vi "Actor Core.vi"(8 "error in":errorcluster, 11 "Monitor Window in":refnum<class "Classic Monitor.lvclass">) -> (0 "error out":errorcluster, 3 "Actor out":refnum<class "Actor.lvclass">)   [LabVIEW 2017, in "MGI-Monitored Actor.lvlib" / "Classic Monitor.lvclass"]
doc: "(<B>Filename</B>: Actor Framework.lvlib:Actor.lvclass:Actor Core.vi)\n\nReceives messages to the actor, reacts to them, and initiates any error handling that may shut the actor down.\n\nDescendant classes may override this VI to append parallel tasks for the actor to complete while it handles messages. Overrides use the Call Parent Method node."
uses:
  Classic Monitor.lvclass
  C:/Program Files (x86)/National Instruments/LabVIEW 2017/vi.lib/ActorFramework/Actor/Actor.lvclass
  <vilib>/ActorFramework/Actor/Actor.lvclass
  monitored-actor-core/Source/Monitor Data/Monitor Data.lvclass
  <vilib>/ActorFramework/Message Enqueuer/Message Enqueuer.lvclass
  <vilib>/ActorFramework/Actor/Actor.lvclass/Actor.ctl
  <vilib>/ActorFramework/Message Enqueuer/Message Enqueuer.lvclass/Message Enqueuer.ctl
  Classic Monitor.lvclass/Classic Monitor.ctl
  <vilib>/ActorFramework/Time-Delayed Send Message/Time-Delay Override Options.ctl
  <vilib>/ActorFramework/Stop Msg/Stop Msg.lvclass/Stop Msg.ctl
  Orphan Detector/Orphan Detector/Orphan Detector.lvclass
  <vilib>/ActorFramework/Message Enqueuer/Init from Existing Queue.vi
  <vilib>/ActorFramework/Message Enqueuer/Enqueue.vi
  <vilib>/ActorFramework/Message Enqueuer/Enqueue Critical.vi
  <vilib>/ActorFramework/Stop Msg/Stop Msg.lvclass
  C:/Program Files (x86)/National Instruments/LabVIEW 2017/vi.lib/ActorFramework/Message/Message.lvclass
  monitored-actor-core/Source/Actor Monitor/Actor Monitor Messages/Ping Actor Msg/Ping Actor Msg.lvclass
  <vilib>/ActorFramework/Message Priority Queue/Priority Enqueue.vi
  monitored-actor-core/Source/Actor Monitor/Actor Monitor/Actor Monitor.lvclass
  Classic Monitor Messages/Log Messages Msg/Log Messages Msg.lvclass
  monitored-actor-core/Source/Actor Monitor/Actor Monitor Messages/Manually Remove Actor Msg/Manually Remove Actor Msg.lvclass
panel:
  in  "Monitored Actors":string[](tree)
  in  "Stop Actor":bool
  in  "Show Actor Core":bool
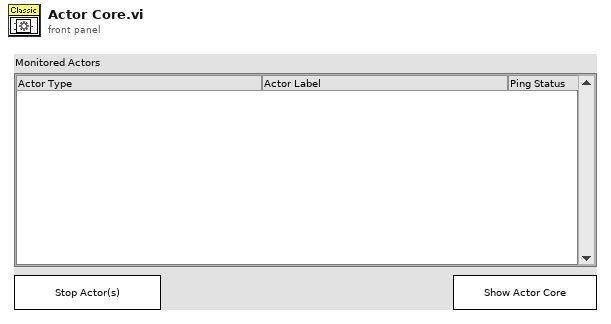
[diagram p1: front panel]
types:
  T1 = cluster{"Monitor Data":refnum<class "Monitor Data.lvclass">, "Changed Actor Q":refnum<class "Message Enqueuer.lvclass">}
  T2 = enum32{"Invalid", "Standard", "Closed", "Hidden", "Minimized", "Maximized"}
  T3 = cluster{"left":i16, "top":i16, "right":i16, "bottom":i16}
  T4 = typedef "Time-Delay Override Options.ctl" = enum16{"Send next copy now", "Skip next scheduled copy", "Send next copy now and stop all further copies", "Stop all further copies"}
  T5 = enum8{"Enabled", "Disabled", "Disabled and Grayed Out"}
  T6 = typedef "LVRectTypeDef.ctl" = cluster{"Left":i16, "Top":i16, "Right":i16, "Bottom":i16}
  T7 = typedef "LVPoint32TypeDef.ctl" = cluster{"Horizontal":i32, "Vertical":i32}
  T8 = typedef "MGI-Monitored Actor Core.lvlib/Monitor Data.lvclass/Actor Data.ctl" = cluster{"Actor Type":string, "Actor Cores":string[], "Self":refnum<class "Message Enqueuer.lvclass">, "Caller":refnum<class "Message Enqueuer.lvclass">, "Actor Label":string, "Last Ping":dbl}
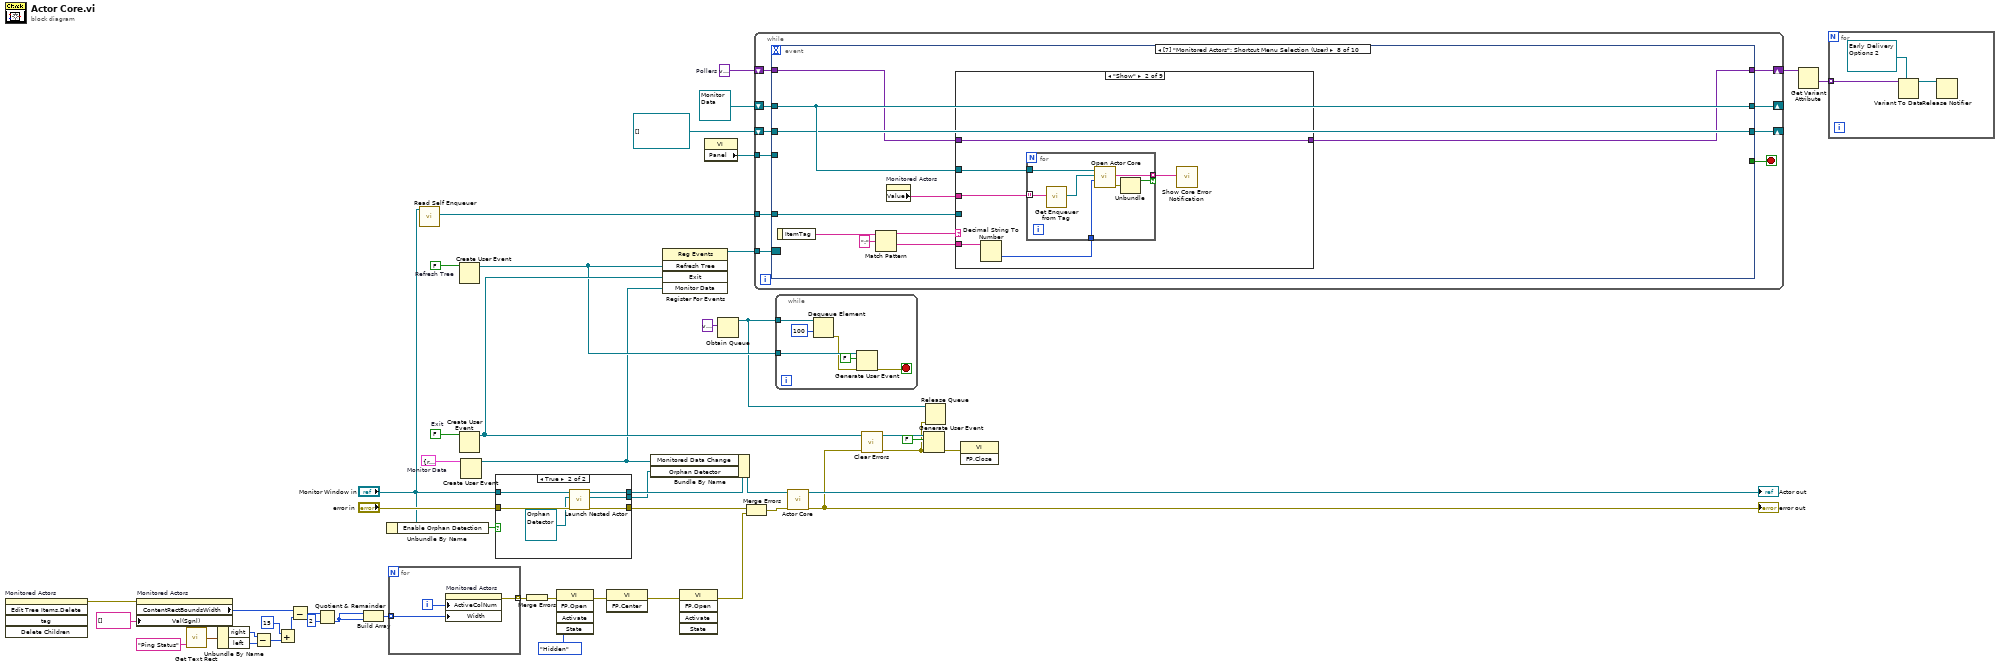
[diagram p0: block diagram]
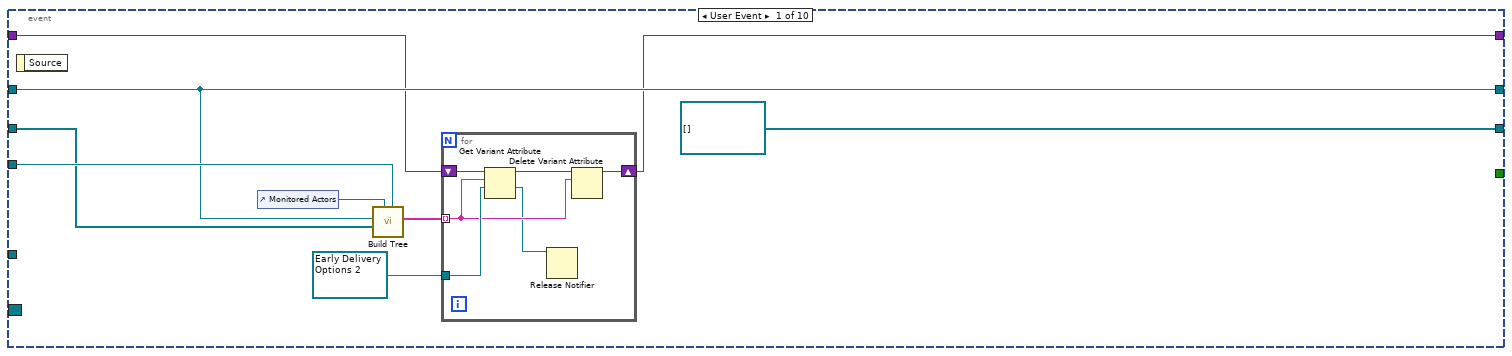
[diagram p3: hidden frame]
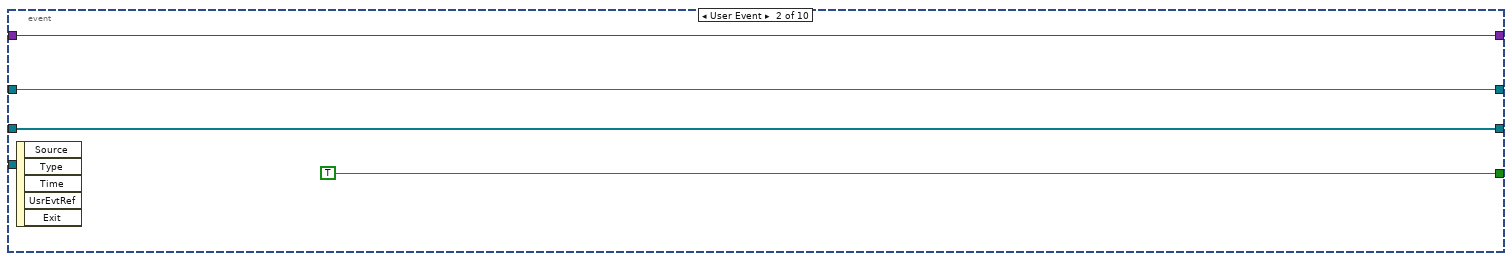
[diagram p4: hidden frame]
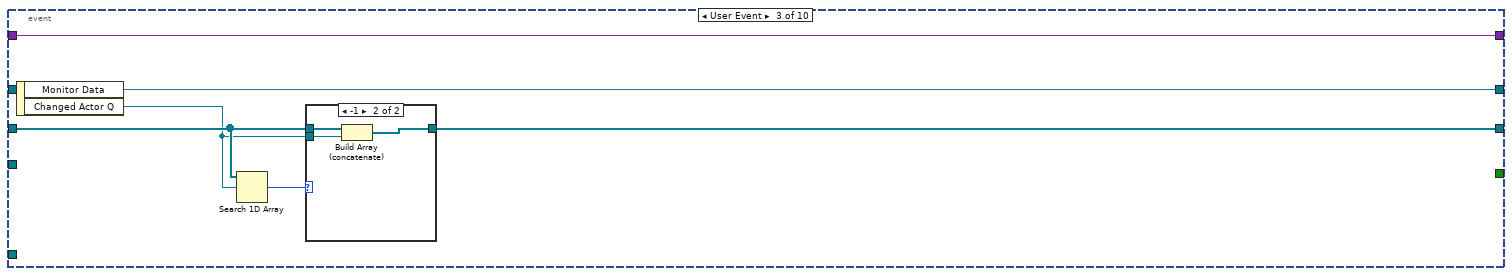
[diagram p5: hidden frame]
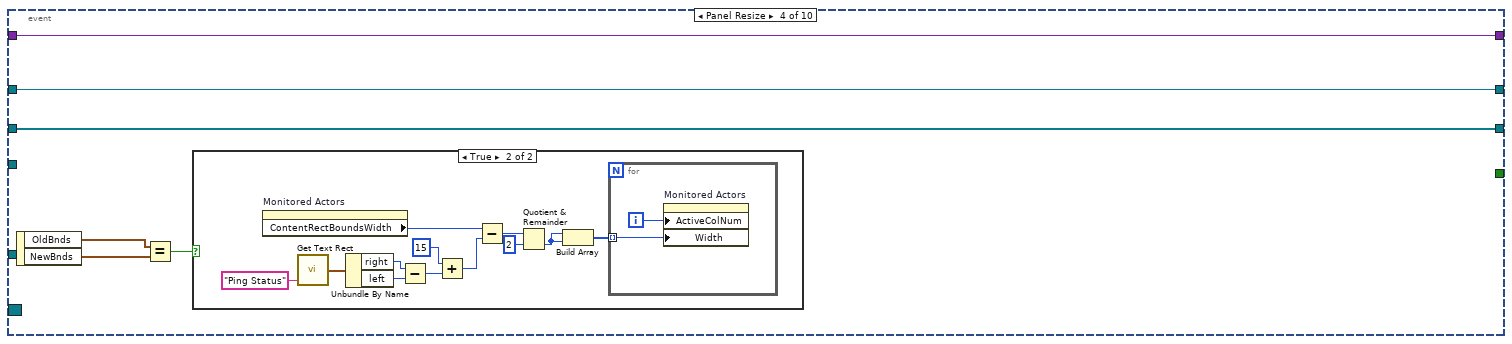
[diagram p7: hidden frame]
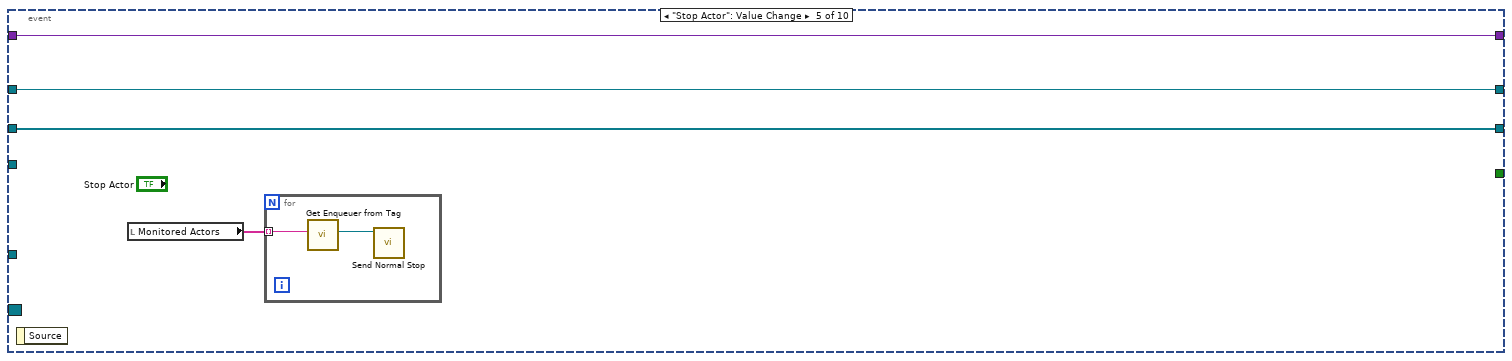
[diagram p9: hidden frame]
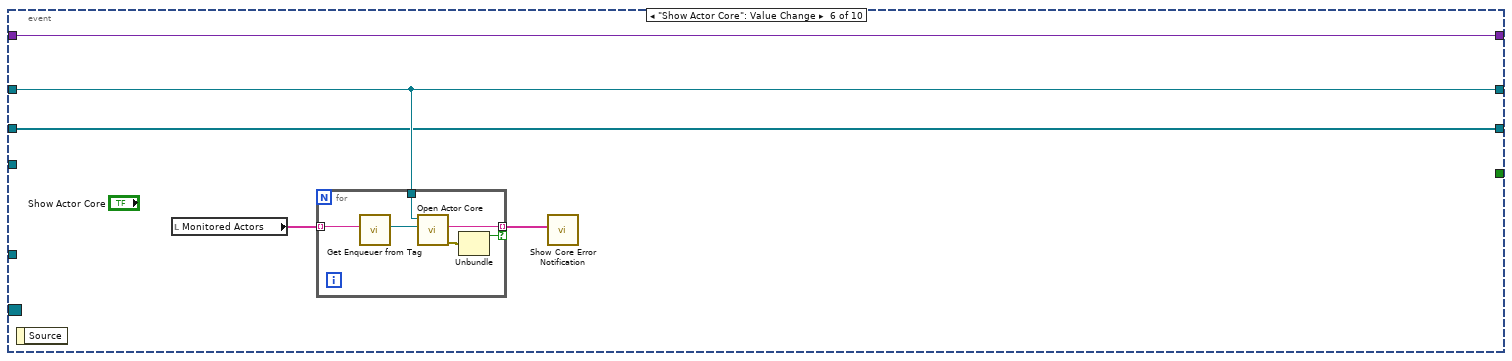
[diagram p10: hidden frame]
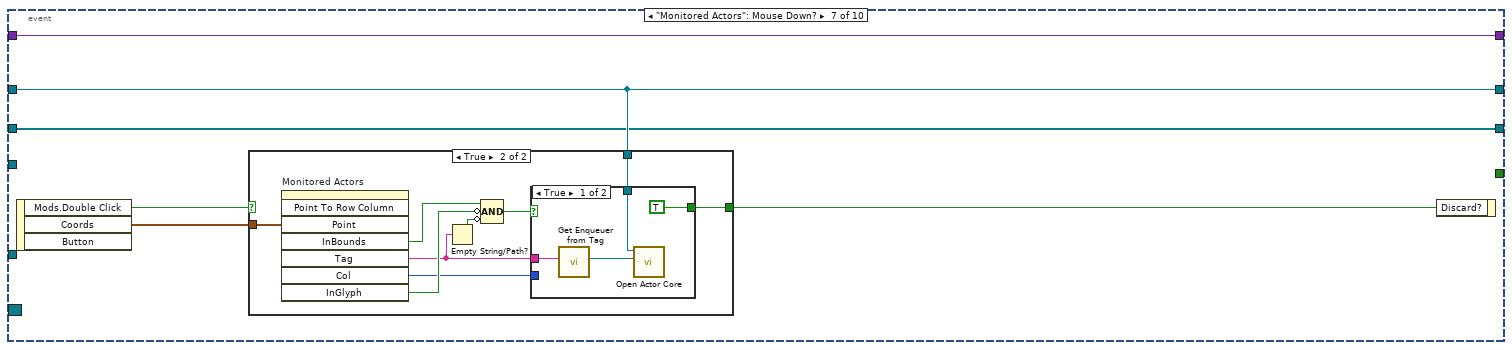
[diagram p11: hidden frame]
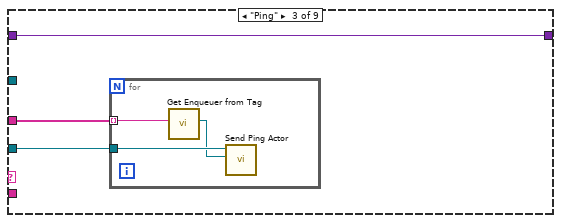
[diagram p15: hidden frame]
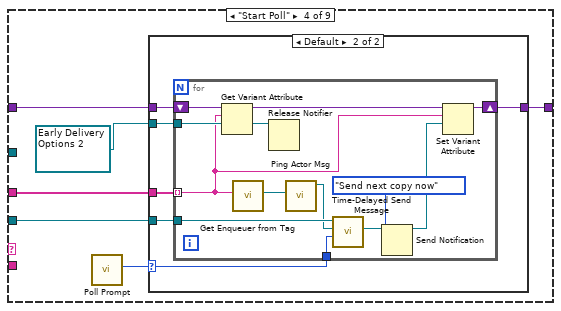
[diagram p16: hidden frame]
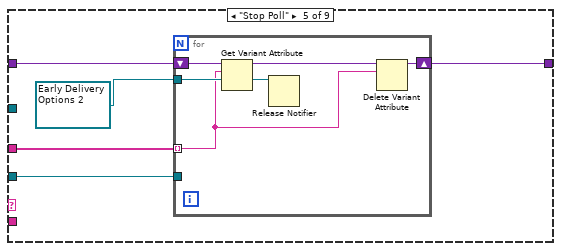
[diagram p18: hidden frame]
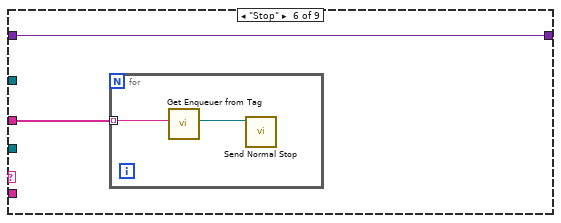
[diagram p19: hidden frame]
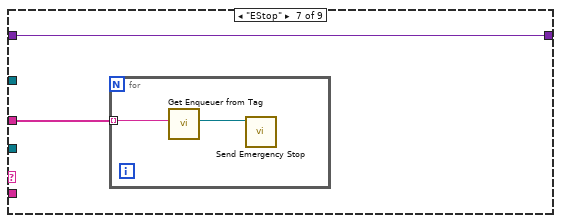
[diagram p20: hidden frame]
diagram:
  w6 = variant  # Pollers
  w17 = T1 {"Monitor Data"=refnum, "Changed Actor Q"=refnum}  # Monitor Data
  w22 = FALSE  # Refresh Tree
  w34 = FALSE  # Exit
  n1 = invoke on="Monitored Actors" class="Tree (strict)" method="Edit Tree Items.Delete"() -> (error out=w13:errorcluster)  [unwired: 5 in, 4 out]
  n2 = property on="Monitored Actors" class="Tree (strict)"(error in=w13, "Val(Sgnl)"=string[] [] ("Value (Signaling)")) -> ("ContentRectBoundsWidth"=w47:i32)  [unwired: 1 in, 2 out]
  n3 = call <vilib>:"Get Text Rect.vi"("text"="Ping Status") -> ("rect"=w45:T3)  [unwired: 8 in]
  n4 = Unbundle By Name(w45) -> ("right"=w44:i16, "left"=w43:i16)
  n5 = Subtract(x=w44, y=w43) -> (x-y=w42:i16)
  n6 = Add(x=i16 15, y=w42) -> (x+y=w39:i16)
  n7 = Subtract(x=w47, y=w39) -> (x-y=w41:i32)
  n8 = Quotient & Remainder(x=w41, y=2) -> (floor(x/y)=w37:i32)  [unwired: 1 out]
  n9 = Build Array(w37, w37) -> (w36:i32[])
  n10 = Unbundle By Name("Monitor Window in") -> ("Enable Orphan Detection"=w7:bool)
  n11 = for {
    tunnel: w36 -> [w51] mode=indexing
    tunnel: [w50] -> w27 mode=indexing
    i -> [w52]
    n12 = property on="Monitored Actors" class="Tree (strict)"("ActiveColNum"=w52, "Width"=w51) -> (error out=w50:errorcluster)  [unwired: 2 in, 1 out]
  }
  n13 = call <vilib>:"Read Self Enqueuer.vi"("Actor"="Monitor Window in") -> ("Self Enqueuer"=w28:refnum<class "Message Enqueuer.lvclass">)  [unwired: 10 in]
  n14 = Create User Event(user event datatype=w22) -> (user event=w21:refnum<user-event>)  [unwired: 1 in, 1 out]
  n15 = Create User Event(user event datatype=w34) -> (user event=w33:refnum<user-event>)  [unwired: 1 in, 1 out]
  n16 = Create User Event(user event datatype=w17) -> (user event=w16:refnum<user-event>)  [unwired: 1 in, 1 out]
  n17 = case shown="True" w7 {
    tunnel: "error in" -> [w53 w56]
    tunnel: [w53 w57] -> w12
    tunnel: [w54 w59] -> w11
    tunnel: "Monitor Window in" -> [w54 w60]
    tunnel: [_ w58] -> w10
    frame False {
    }
    frame True {
      n18 = call <vilib>:"Launch Nested Actor.vi"("error in (no error)"=w56, "Nested Actor"=refnum<class "Orphan Detector.lvclass"> refnum ("Classic Monitor.lvlib:Orphan Detector.lvclass"), "Caller Actor in"=w60) -> ("error out"=w57:errorcluster, "Nested Actor's Enqueuer"=w58:refnum<class "Message Enqueuer.lvclass">, "Caller Actor out"=w59:refnum<class "Classic Monitor.lvclass">)  [unwired: 6 in]
    }
  }
  n19 = Merge Errors(w27) -> (w25:errorcluster)
  n20 = invoke class="VI" method="FP.Open"(error in=w25, "State"=T2."Hidden") -> (error out=w26:errorcluster)  [unwired: 3 in, 4 out]
  n21 = invoke class="VI" method="FP.Center"(error in=w26) -> (error out=w24:errorcluster)  [unwired: 2 in, 2 out]
  n22 = Bundle By Name(cluster=w11, "Monitored Data Change"=w16, "Orphan Detector"=w10) -> (w31:refnum<class "Classic Monitor.lvclass">)
  n23 = register-events(w21, w33, w16) -> (reference out=w35:refnum<event-registration>)  [unwired: 2 in, 1 out]
  n24 = invoke class="VI" method="FP.Open"(error in=w24) -> (error out=w1:errorcluster)  [unwired: 4 in, 4 out]
  n25 = property class="VI"() -> ("Panel"=w29:refnum<vi>)  [unwired: 2 in, 2 out]
  n26 = Obtain Queue(element data type=variant) -> (queue out=w18:refnum<queue>)  [unwired: 4 in, 2 out]
  n27 = Merge Errors(w12, w1) -> (w2:errorcluster)
  n28 = while {
    tunnel: w35 -> [w70]
    shift-right: [w68] -> _
    shift-left: refnum<class "Monitor Data.lvclass"> refnum ("Monitor Data") -> [w67]
    tunnel: w29 -> [w66]
    tunnel: w28 -> [w65]
    shift-right: [w64] -> _
    shift-left: refnum<class "Message Enqueuer.lvclass">[] [] -> [w63]
    shift-right: [w62] -> w5
    shift-left: w6 -> [w61]
    stop <- w69 stop-if-true
    n29 = event shown="[7] \"Monitored Actors\": Shortcut Menu Selection (User)" {
      selector: w70 -> [_ _ _ _ _ _ _ _ _ _]
      dyn-events: _ -> [_ _ _ _ _ _ _ _ _ _]
      timeout: _ -> [_ _ _ _ _ _ _ _ _ _]
      tunnel: [_ TRUE _ _ _ _ _ _ _ _] -> w69
      tunnel: [w78 w88 w95 w105 w123 w129 w142 w165 w253 w255] -> w68
      tunnel: w67 -> [w78 w88 _ w105 w123 w129 w142 w165 w253 w255]
      tunnel: w66 -> [w79 _ _ _ _ _ _ _ _ _]
      tunnel: w65 -> [_ _ _ _ _ _ _ w163 _ _]
      tunnel: [refnum<class "Message Enqueuer.lvclass">[] [] w87 w94 w101 w121 w128 w138 w162 w254 w276] -> w64
      tunnel: w63 -> [w76 w87 w93 w101 w121 w128 w138 w162 w254 w276]
      tunnel: [w71 w86 w90 w100 w120 w126 w137 w160 w247 w269] -> w62
      tunnel: w61 -> [w72 w86 w90 w100 w120 w126 w137 w161 w247 w269]
      event User Event {
        w73 = refnum<notifier> refnum items=["Send next copy now", "Skip next scheduled copy", "Send next copy now and stop all further copies", "Stop all further copies"] ("Delivery Notifier")
        n30 = event-data() -> ()  [unwired: 1 in, 1 out]
        n31 = control-ref of="Monitored Actors"() -> (w77:refnum<vi>)
        n32 = call "Build Tree.vi"("Panel"=w79, "Tree"=w77, "Changed Actors"=w76, "Monitor Data"=w78) -> ("Stopped Actors"=w74:string[])  [unwired: 7 in]
        n33 = for {
          tunnel: w74 -> [w82] mode=indexing
          shift-right: [w81] -> w71
          shift-left: w72 -> [w85]
          tunnel: w73 -> [w84]
          n34 = Get Variant Attribute(Variant=w85, name=w82, default value (empty Variant)=w84) -> (duplicate Variant=w83:variant, value=w80:refnum<notifier>)  [unwired: 1 in, 2 out]
          n35 = Release Notifier(notifier=w80) -> ()  [unwired: 2 in, 3 out]
          n36 = Delete Variant Attribute(6:w82, 7:w83) -> (3:w81:variant)  [unwired: 1 in, 2 out]
        }
      }
      event User Event {
        n37 = event-data() -> ()  [unwired: 1 in, 5 out]
      }
      event User Event {
        n38 = event-data() -> ("Monitor Data"=w95:refnum<class "Monitor Data.lvclass">, "Changed Actor Q"=w92:refnum<class "Message Enqueuer.lvclass">)  [unwired: 1 in]
        n39 = Search 1D Array(1D array=w93, element=w92) -> (index of element=w91:i32)  [unwired: 1 in]
        n40 = case shown="-1" w91 {
          tunnel: [w96 w99] -> w94
          tunnel: w93 -> [w96 w98]
          tunnel: w92 -> [_ w97]
          frame Default {
          }
          frame -1 {
            n41 = Build Array (concatenate)(w98, w97) -> (w99:refnum<class "Message Enqueuer.lvclass">[])
          }
        }
      }
      event Panel Resize {
        n42 = event-data() -> ("OldBnds"=w104:T6, "NewBnds"=w103:T6)  [unwired: 1 in]
        n43 = Equal?(x=w104, y=w103) -> (x = y?=w102:bool)
        n44 = case shown="True" w102 {
          frame False {
          }
          frame True {
            n45 = property on="Monitored Actors" class="Tree (strict)"() -> ("ContentRectBoundsWidth"=w106:i32)  [unwired: 2 in, 2 out]
            n46 = call <vilib>:"Get Text Rect.vi"("text"="Ping Status") -> ("rect"=w108:T3)  [unwired: 8 in]
            n47 = Unbundle By Name(w108) -> ("right"=w109:i16, "left"=w110:i16)
            n48 = Subtract(x=w109, y=w110) -> (x-y=w111:i16)
            n49 = Add(x=i16 15, y=w111) -> (x+y=w114:i16)
            n50 = Subtract(x=w106, y=w114) -> (x-y=w112:i32)
            n51 = Quotient & Remainder(x=w112, y=2) -> (floor(x/y)=w116:i32)  [unwired: 1 out]
            n52 = Build Array(w116, w116) -> (w117:i32[])
            n53 = for {
              tunnel: w117 -> [w118] mode=indexing
              i -> [w119]
              n54 = property on="Monitored Actors" class="Tree (strict)"("ActiveColNum"=w119, "Width"=w118) -> ()  [unwired: 2 in, 2 out]
            }
          }
        }
      }
      event "Stop Actor": Value Change {
        n55 = event-data() -> ()  [unwired: 1 in, 1 out]
        n56 = local read "Monitored Actors"() -> (w122:string[])
        n57 = for {
          tunnel: w122 -> [w125] mode=indexing
          n58 = call "Get Enqueuer from Tag.vi"("Tag"=w125) -> ("Enqueuer"=w124:refnum<class "Message Enqueuer.lvclass">)  [unwired: 10 in]
          n59 = call <vilib>:"Send Normal Stop.vi"("Message Enqueuer"=w124) -> ()  [unwired: 10 in, 1 out]
        }
      }
      event "Show Actor Core": Value Change {
        n60 = event-data() -> ()  [unwired: 1 in, 1 out]
        n61 = local read "Monitored Actors"() -> (w130:string[])
        n62 = for {
          tunnel: w130 -> [w136] mode=indexing
          tunnel: w129 -> [w135]
          tunnel: [w133] -> w127 mode=indexing if=w131
          n63 = call "Get Enqueuer from Tag.vi"("Tag"=w136) -> ("Enqueuer"=w134:refnum<class "Message Enqueuer.lvclass">)  [unwired: 10 in]
          n64 = call "Open Actor Core.vi"("Actor's Self Q"=w134, "Monitor Data"=w135) -> ("error out"=w132:errorcluster, "Actor Core VI"=w133:string)  [unwired: 8 in]
          n65 = Unbundle(w132) -> ("status"=w131:bool)  [unwired: 2 out]
        }
        n66 = call "Show Core Error Notification.vi"("Error VIs"=w127) -> ()  [unwired: 11 in]
      }
      event "Monitored Actors": Mouse Down? {
        n67 = event-data() -> ("Mods.Double Click"=w141:bool, "Coords"=w140:T7)  [unwired: 1 in, 1 out]
        n68 = case shown="True" w141 {
          tunnel: w142 -> [_ w151]
          tunnel: w140 -> [_ w150]
          tunnel: [_ w147] -> w139
          frame False {
          }
          frame True {
            n69 = invoke on="Monitored Actors" class="Tree (strict)" method="Point To Row Column"("Point"=w150) -> ("InBounds"=w149:bool, "Tag"=w144:string, "Col"=w143:i32, "InGlyph"=w148:bool)  [unwired: 7 in, 4 out]
            n70 = Empty String/Path?(string/path=w144) -> (empty?=w145:bool)
            n71 = Compound Arithmetic op=AND(w149, invert w148, invert w145) -> (w146:bool)
            n72 = case shown="True" w146 {
              tunnel: w151 -> [w153 _]
              tunnel: [TRUE _] -> w147
              tunnel: w144 -> [w155 _]
              tunnel: w143 -> [_ _]
              frame True {
                n73 = call "Get Enqueuer from Tag.vi"("Tag"=w155) -> ("Enqueuer"=w152:refnum<class "Message Enqueuer.lvclass">)  [unwired: 10 in]
                n74 = call "Open Actor Core.vi"("Actor's Self Q"=w152, "Monitor Data"=w153) -> ()  [unwired: 8 in, 2 out]
              }
              frame False {
              }
            }
          }
        }
        n75 = event-data("Discard?"=w139) -> ()  [unwired: 1 in, 1 out]
      }
      event "Monitored Actors": Shortcut Menu Selection (User) {
        n76 = event-data() -> ("ItemTag"=w159:string)  [unwired: 1 in]
        n77 = Match Pattern(string=w159, regular expression=":") -> (before substring=w158:string, after substring=w156:string)  [unwired: 1 in, 2 out]
        n78 = property on="Monitored Actors" class="Tree (strict)"() -> ("Value"=w164:string[])  [unwired: 2 in, 2 out]
        n79 = case shown="\"Show\"" w158 {
          tunnel: w165 -> [_ w171 _ _ _ _ _ _ _]
          tunnel: w164 -> [_ w172 w182 w191 w216 w224 w228 w235 w243]
          tunnel: w163 -> [_ _ w181 w190 w215 _ _ w234 w242]
          tunnel: w161 -> [w166 w169 w180 w189 w214 w223 w227 w233 w241]
          tunnel: [w166 w169 w180 w188 w213 w223 w227 w233 w241] -> w160
          tunnel: w156 -> [_ w168 _ _ _ _ _ _ _]
          frame Default {
          }
          frame "Show" {
            n80 = Decimal String To Number(string=w168) -> (number=w167:i32)  [unwired: 2 in, 1 out]
            n81 = for {
              tunnel: w172 -> [w179] mode=indexing
              tunnel: w171 -> [w178]
              tunnel: [w176] -> w170 mode=indexing if=w174
              tunnel: w167 -> [w173]
              n82 = call "Get Enqueuer from Tag.vi"("Tag"=w179) -> ("Enqueuer"=w177:refnum<class "Message Enqueuer.lvclass">)  [unwired: 10 in]
              n83 = call "Open Actor Core.vi"("Core Index (0)"=w173, "Actor's Self Q"=w177, "Monitor Data"=w178) -> ("error out"=w175:errorcluster, "Actor Core VI"=w176:string)  [unwired: 7 in]
              n84 = Unbundle(w175) -> ("status"=w174:bool)  [unwired: 2 out]
            }
            n85 = call "Show Core Error Notification.vi"("Error VIs"=w170) -> ()  [unwired: 11 in]
          }
          frame "Ping" {
            n86 = for {
              tunnel: w182 -> [w185] mode=indexing
              tunnel: w181 -> [w184]
              n87 = call "Get Enqueuer from Tag.vi"("Tag"=w185) -> ("Enqueuer"=w183:refnum<class "Message Enqueuer.lvclass">)  [unwired: 10 in]
              n88 = call "Send Ping Actor.vi"("Actor"=w183, "Message Enqueuer in"=w184) -> ()  [unwired: 8 in, 2 out]
            }
          }
          frame "Start Poll" {
            w187 = refnum<notifier> refnum items=["Send next copy now", "Skip next scheduled copy", "Send next copy now and stop all further copies", "Stop all further copies"] ("Delivery Notifier")
            n89 = call "Poll Prompt.vi"() -> ("Period"=w186:i32)  [unwired: 10 in, 1 out]
            n90 = case shown="Default" w186 {
              selector: w186 -> [_ w193]
              tunnel: w191 -> [_ w198]
              tunnel: w190 -> [_ w197]
              tunnel: w189 -> [w192 w196]
              tunnel: [w192 w195] -> w188
              tunnel: w187 -> [_ w194]
              frame -1 {
              }
              frame Default {
                n91 = for {
                  tunnel: w198 -> [w202] mode=indexing
                  tunnel: w197 -> [w211]
                  shift-right: [w204] -> w195
                  shift-left: w196 -> [w208]
                  tunnel: w194 -> [w206]
                  tunnel: w193 -> [w201]
                  n92 = Get Variant Attribute(Variant=w208, name=w202, default value (empty Variant)=w206) -> (duplicate Variant=w207:variant, value=w205:refnum<notifier>)  [unwired: 1 in, 2 out]
                  n93 = call "Get Enqueuer from Tag.vi"("Tag"=w202) -> ("Enqueuer"=w210:refnum<class "Message Enqueuer.lvclass">)  [unwired: 10 in]
                  n94 = Release Notifier(notifier=w205) -> ()  [unwired: 2 in, 3 out]
                  n95 = call "Ping Actor Msg.vi"("Actor"=w210) -> ("Ping Actor Msg out"=w209:refnum<class "Ping Actor Msg.lvclass">)  [unwired: 9 in, 1 out]
                  n96 = call <vilib>:"Time-Delayed Send Message.vi"("Milliseconds To Wait"=w201, "Message"=w209, "Message Enqueuer"=w211) -> ("Delivery Notifier"=w203:refnum<notifier>)  [unwired: 7 in, 1 out]
                  n97 = Send Notification(notification=Time-Delay_Override_Options."Send next copy now", notifier=w203) -> (notifier out=w200:refnum<notifier>)  [unwired: 1 in, 1 out]
                  n98 = Set Variant Attribute(Variant=w207, name=w202, value=w200) -> (Variant out=w204:variant)  [unwired: 1 in, 2 out]
                }
              }
            }
          }
          frame "Stop Poll" {
            w212 = refnum<notifier> refnum items=["Send next copy now", "Skip next scheduled copy", "Send next copy now and stop all further copies", "Stop all further copies"] ("Delivery Notifier")
            n99 = for {
              tunnel: w216 -> [w217] mode=indexing
              tunnel: w215 -> [_]
              shift-right: [w218] -> w213
              shift-left: w214 -> [w222]
              tunnel: w212 -> [w220]
              n100 = Get Variant Attribute(Variant=w222, name=w217, default value (empty Variant)=w220) -> (duplicate Variant=w221:variant, value=w219:refnum<notifier>)  [unwired: 1 in, 2 out]
              n101 = Release Notifier(notifier=w219) -> ()  [unwired: 2 in, 3 out]
              n102 = Delete Variant Attribute(6:w217, 7:w221) -> (3:w218:variant)  [unwired: 1 in, 2 out]
            }
          }
          frame "Stop" {
            n103 = for {
              tunnel: w224 -> [w226] mode=indexing
              n104 = call "Get Enqueuer from Tag.vi"("Tag"=w226) -> ("Enqueuer"=w225:refnum<class "Message Enqueuer.lvclass">)  [unwired: 10 in]
              n105 = call <vilib>:"Send Normal Stop.vi"("Message Enqueuer"=w225) -> ()  [unwired: 10 in, 1 out]
            }
          }
          frame "EStop" {
            n106 = for {
              tunnel: w228 -> [w230] mode=indexing
              n107 = call "Get Enqueuer from Tag.vi"("Tag"=w230) -> ("Enqueuer"=w229:refnum<class "Message Enqueuer.lvclass">)  [unwired: 10 in]
              n108 = call <vilib>:"Send Emergency Stop.vi"("Message Enqueuer"=w229) -> ()  [unwired: 10 in, 1 out]
            }
          }
          frame "Remove" {
            n109 = Two Button Dialog(message="Warning: Manually removing actors from list can lead to inconsitancies between the monitor and the actual state.\n\n Only do this if you're sure the actor has been aborted manually.") -> (T button?=w231:bool)  [unwired: 2 in]
            n110 = case shown="True" w231 {
              tunnel: w235 -> [_ w237]
              tunnel: w234 -> [_ w236]
              frame False {
              }
              frame True {
                n111 = for {
                  tunnel: w237 -> [w240] mode=indexing
                  tunnel: w236 -> [w238]
                  n112 = call "Get Enqueuer from Tag.vi"("Tag"=w240) -> ("Enqueuer"=w239:refnum<class "Message Enqueuer.lvclass">)  [unwired: 10 in]
                  n113 = call "Send Manually Remove Actor.vi"("Actor's Q"=w239, "Message Enqueuer in"=w238) -> ()  [unwired: 8 in, 2 out]
                }
              }
            }
          }
          frame "Logging" {
            n114 = for {
              tunnel: w243 -> [w246] mode=indexing
              tunnel: w242 -> [w245]
              n115 = call "Get Enqueuer from Tag.vi"("Tag"=w246) -> ("Enqueuer"=w244:refnum<class "Message Enqueuer.lvclass">)  [unwired: 10 in]
              n116 = call "Send Log Messages.vi"("Actor to Log"=w244, "Message Enqueuer in"=w245) -> ()  [unwired: 8 in, 2 out]
            }
          }
        }
      }
      event "Monitored Actors": Value Change {
        n117 = event-data() -> ()  [unwired: 1 in, 1 out]
        n118 = Empty Array?(array="Monitored Actors") -> (empty?=w251:bool)
        n119 = Select(t=T5."Disabled and Grayed Out" ("Disabled"), s=w251, f=T5."Enabled") -> (s? t:f=w248:T5)
        n120 = property on="Stop Actor" class="Bool"("DisabledEnum"=w248) -> ()  [unwired: 2 in, 2 out]
        n121 = property on="Show Actor Core" class="Bool"("DisabledEnum"=w248) -> ()  [unwired: 2 in, 2 out]
      }
      event "Monitored Actors": Shortcut Menu Activation? {
        w258 = "Show" ("item tag")
        n122 = event-data() -> ("MenuRef"=w275:refnum<k9>, "Coords"=w274:T7)  [unwired: 1 in]
        n123 = invoke on="Monitored Actors" class="Tree (strict)" method="Point To Row Column"("Point"=w274) -> ("Tag"=w273:string)  [unwired: 7 in, 7 out]
        n124 = disable-structure shown="Disable_Msg_Log==True" {
          disable-tunnel: w275 -> [w298 w299]
          disable-tunnel: [w295 w299] -> w267
          frame condition #0 {
            n125 = Set Menu Item Info(7:"Logging" ("item name"), 9:FALSE ("enabled"), 11:w298) -> (3:w295:refnum<k9>)  [unwired: 4 in, 1 out]
          }
          frame condition #1 (active) {
          }
        }
        n126 = property on="Monitored Actors" class="Tree (strict)"() -> ("Value"=w270:string[])  [unwired: 2 in, 2 out]
        n127 = Search 1D Array(1D array=w270, element=w273) -> (index of element=w271:i32)  [unwired: 1 in]
        n128 = Build Array(w273) -> (w272:string[])
        n129 = case shown="Default" w271 {
          tunnel: w272 -> [_ w294]
          tunnel: w270 -> [w292 w293]
          tunnel: [w292 w293] -> w256
          frame Default {
          }
          frame -1 {
            n130 = property on="Monitored Actors" class="Tree (strict)"("Val(Sgnl)"=w294) -> ()  [unwired: 2 in, 2 out]
          }
        }
        n131 = for {
          tunnel: w256 -> [w290] mode=indexing
          tunnel: w269 -> [w291]
          tunnel: [w289] -> w264 mode=indexing
          n132 = Get Variant Attribute(Variant=w291, name=w290) -> (found=w289:bool)  [unwired: 2 in, 3 out]
        }
        n133 = Array Size(array=w256) -> (size(s)=w257:i32)
        n134 = Or Array Elements(Boolean array=w264) -> (logical OR=w261:bool)
        n135 = And Array Elements(Boolean array=w264) -> (logical AND=w263:bool)
        n136 = Not(x=w263) -> (.not. x?=w262:bool)
        n137 = Set Menu Item Info(7:"Stop Poll" ("item name"), 9:w261, 11:w267) -> (3:w266:refnum<k9>)  [unwired: 4 in, 1 out]
        n138 = Set Menu Item Info(7:"Start Poll" ("item tag"), 9:w262, 11:w266) -> (3:w260:refnum<k9>)  [unwired: 4 in, 1 out]
        n139 = Delete Menu Items(8:w258, 9:w260) -> (3:w259:refnum<k9>)  [unwired: 2 in, 1 out]
        n140 = case shown="1" w257 {
          tunnel: w259 -> [_ w285]
          tunnel: w258 -> [_ w284]
          tunnel: w256 -> [_ w283]
          tunnel: w255 -> [_ w281]
          frame Default {
          }
          frame 1 {
            n141 = Index Array(array=w283) -> (element=w282:string)  [unwired: 1 in]
            n142 = call "Get Enqueuer from Tag.vi"("Tag"=w282) -> ("Enqueuer"=w280:refnum<class "Message Enqueuer.lvclass">)  [unwired: 10 in]
            n143 = call "Get Actor Data.vi"("Actor's Self Q"=w280, "Monitor Data in"=w281) -> ("Actor Data"=w279:T8)  [unwired: 6 in, 3 out]
            n144 = Unbundle By Name(w279) -> ("Actor Cores"=w278:string[])
            n145 = for {
              tunnel: w278 -> [_] mode=indexing
              tunnel: [w286] -> w277 mode=indexing
              i -> [w288]
              n146 = Format Into String(format string="Show:%d", w288) -> (resulting string=w286:string)  [unwired: 2 in, 1 out]
            }
            n147 = Insert Menu Items(5:w284, 7:w277, 8:w278, 9:w285) -> ()  [unwired: 2 in, 3 out]
          }
        }
        n148 = event-data() -> ()  [unwired: 2 in, 1 out]
      }
    }
  }
  n149 = while {
    tunnel: w18 -> [w304]
    tunnel: w21 -> [w303]
    stop <- w301 stop-if-true
    n150 = Dequeue Element(queue=w304, timeout in ms (-1)=100) -> (error out=w302:errorcluster)  [unwired: 1 in, 3 out]
    n151 = Generate User Event(user event=w303, event data cluster=FALSE ("event data"), error in=w302) -> (error out=w301:errorcluster)  [unwired: 1 in, 1 out]
  }
  n152 = call-parent "Actor Core.vi"("error in"=w2, "Actor in"=w31) -> ("error out"=w32:errorcluster, "Actor out"=→"Actor out":refnum<class "Actor.lvclass">)  [unwired: 8 in]
  "error out" <- w32
  n153 = call <vilib>:"Clear Errors.vi"("error in (no error)"=w32) -> ("error out"=w19:errorcluster)  [unwired: 5 in, 1 out]
  n154 = Generate User Event(user event=w33, event data cluster=FALSE ("event data"), error in=w19) -> (error out=w3:errorcluster)  [unwired: 1 in, 1 out]
  n155 = Release Queue(queue=w18, error in (no error)=w19) -> ()  [unwired: 1 in, 3 out]
  n156 = invoke class="VI" method="FP.Close"(error in=w3) -> ()  [unwired: 2 in, 3 out]
  n157 = Get Variant Attribute(Variant=w5) -> (values=w4:variant[])  [unwired: 3 in, 3 out]
  n158 = for {
    tunnel: w4 -> [w308] mode=indexing
    w307 = refnum<notifier> refnum items=["Send next copy now", "Skip next scheduled copy", "Send next copy now and stop all further copies", "Stop all further copies"] ("Delivery Notifier")
    n159 = Variant To Data(type=w307, Variant=w308) -> (data=w306:refnum<notifier>)  [unwired: 1 in, 1 out]
    n160 = Release Notifier(notifier=w306) -> ()  [unwired: 2 in, 3 out]
  }
